vi "SPC_get_adjust_parameters.vi"(8 "Error In":errorcluster, 10 "Module No":i16 min=0 max=7 step=1, 11 "DLL Path":path) -> (0 "Error Out":errorcluster, 2 "Module No":i16 min=0 max=7 step=1, 3 "DLL Path":path, 4 "SPC adjust parameters":T1={"vrt1"=64, "vrt2"=128, "vrt3"=192, "dith_g"=128, "gain_1"=1.0, "gain_2"=1.0, "gain_4"=1.0, "gain_8"=1.0, "tac_r0"=1.0, "tac_r1"=1.0, "tac_r2"=1.0, "tac_r4"=1.0, "tac_r8"=1.0, "sync_div"=0} {"sync_div" min=0 max=2; "tac_r8" format="%.2f"; "tac_r4" format="%.2f"; "tac_r2" format="%.2f"; "tac_r1" format="%.2f"; "tac_r0" format="%.2f"; "gain_8" format="%.2f"; "gain_4" format="%.2f"; "gain_2" format="%.2f"; "gain_1" format="%.2f"})   [LabVIEW 2017]
doc: "The structure 'adjpara' is filled with adjust parameters of the SPC module ‘mod_no’ that are \ncurrently in use. The parameters can either be previously loaded from the EEPROM by SPC_init or SPC_get_eeprom_data or - not recommended - set by SPC_set_adust_parameters.\nThe structure \"SPC_Adjust_Para\" is defined in the file spcm_def.h.\nNormally, the adjust parameters need not be read explicitly because the EEPROM is read during SPC_init and the adjust values are taken into account when the SPC module registers \nare loaded.\n\ninfo@becker-hickl.com"
uses:
  SPC_Controls/SPC_adjust_para.ctl
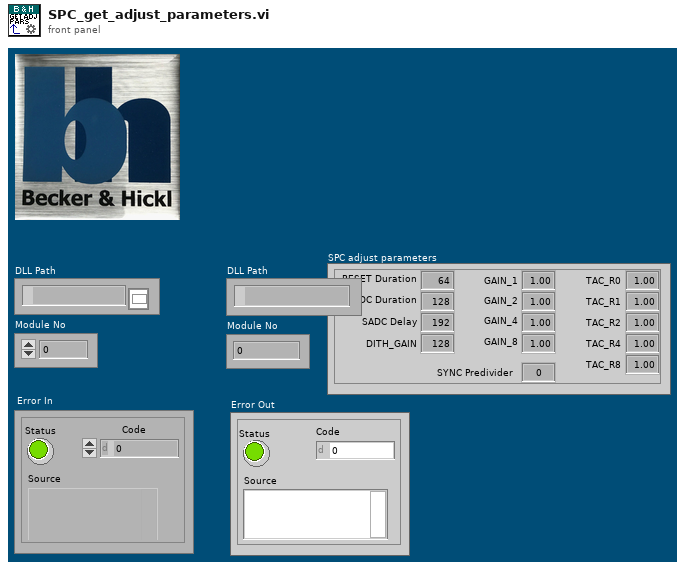
[diagram p1: front panel]
types:
  T1 = typedef "SPC_adjust_para.ctl" = cluster{"vrt1":i16, "vrt2":i16, "vrt3":i16, "dith_g":i16, "gain_1":sgl, "gain_2":sgl, "gain_4":sgl, "gain_8":sgl, "tac_r0":sgl, "tac_r1":sgl, "tac_r2":sgl, "tac_r4":sgl, "tac_r8":sgl, "sync_div":i16}
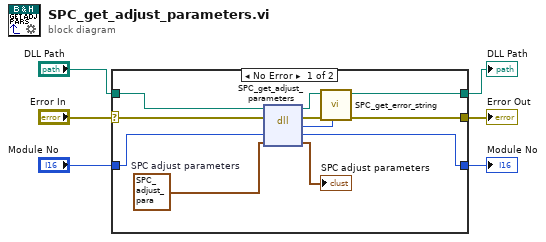
[diagram p0: block diagram]
diagram:
  n1 = case shown="No Error" "Error In" {
    selector: "Error In" -> [w14 w19]
    tunnel: "DLL Path" -> [w16 w20]
    tunnel: [w15 w19] -> w5
    tunnel: [w11 w20] -> w4
    tunnel: "Module No" -> [w10 w18]
    tunnel: [w9 w18] -> w1
    frame No Error {
      w8 = T1 {"vrt1"=64, "vrt2"=128, "vrt3"=192, "dith_g"=128, "gain_1"=1.0, "gain_2"=1.0, "gain_4"=1.0, "gain_8"=1.0, "tac_r0"=1.0, "tac_r1"=1.0, "tac_r2"=1.0, "tac_r4"=1.0, "tac_r8"=1.0, "sync_div"=0}  # SPC adjust parameters
      n2 = dll-call lib="D:/spcm/lib/lab_view/lv10.0/spcm32.dll" fn="SPC_get_adjust_parameters"(path in=w16, error in=w14, "mod_no"=w10, "arg2"=w8) -> (path out=w12:path, error out=w17:errorcluster, "return type"=w13:i16, "mod_no"=w9:i16, "arg2"=→"SPC adjust parameters":T1)  [unwired: 1 in]
      n3 = call "SPC_get_error_string.vi"("ErrorID"=w13, "Error In"=w17, "DLL Path"=w12) -> ("Error Out"=w15:errorcluster, "DLL Path"=w11:path)  [unwired: 6 in, 1 out]
    }
    frame Error {
    }
  }
  "Error Out" <- w5
  "DLL Path" <- w4
  "Module No" <- w1
